vi "move and read QPD.vi"(7 "new position":dbl, 8 "error in":errorcluster, 10 "handle in":i32, 11 "data":dbl[](array[numeric]) format="%0.2f") -> (0 "error out":errorcluster, 2 "handle out":i32, 4 "QPD SD":dbl, 5 "position out":dbl, 6 "QPD mean":dbl)   [LabVIEW 2019]
uses:
  <vilib>/Analysis/NI_AALBase.lvlib
  controller/SubVIs_nanostage/Madlib.dll
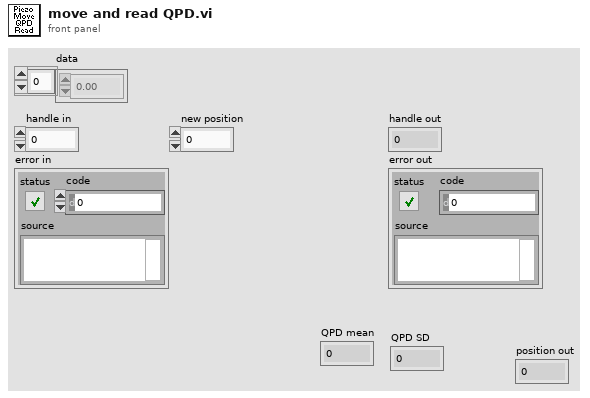
[diagram p1: front panel]
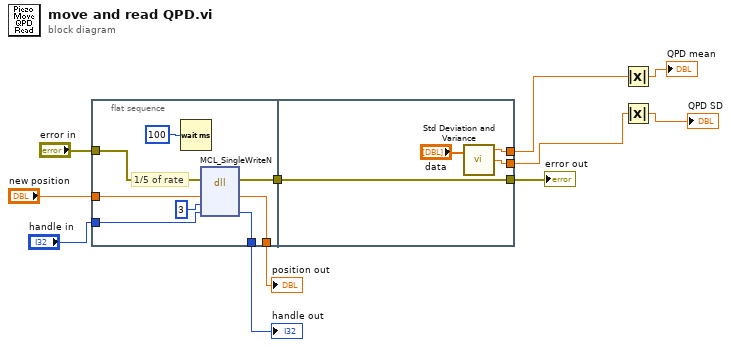
[diagram p0: block diagram]
diagram:
  n1 = flat-sequence {
    tunnel: "handle in" -> [w18]
    tunnel: [w14] -> w11
    tunnel: [w16] -> w9
    tunnel: "error in" -> [w19]
    tunnel: [w15] -> w7
    tunnel: "new position" -> [w13]
    tunnel: w7 -> [w20]
    tunnel: [w20] -> w5
    tunnel: [w23] -> w4
    tunnel: [w22] -> w2
    frame #0 {
      # "1/5 of rate"
      n2 = Wait (ms)(milliseconds to wait=u32 100) -> ()  [unwired: 1 out]
      n3 = dll-call lib="C:/Users/admin/Desktop/controller/SubVIs_nanostage/MADLib.dll" fn="MCL_SingleWriteN"(error in=w19, "position"=w13, "axis"=3, "handle"=w18) -> (error out=w15:errorcluster, "position"=w14:dbl, "handle"=w16:i32)  [unwired: 4 in, 1 out]
    }
    frame #1 {
      n4 = call <vilib>:"Std Deviation and Variance.vi"("X"="data") -> ("mean"=w23:dbl, "standard deviation"=w22:dbl)  [unwired: 1 in, 1 out]
    }
  }
  n5 = Absolute Value(x=w4) -> (abs(x)=→"QPD mean":dbl)
  n6 = Absolute Value(x=w2) -> (abs(x)=→"QPD SD":dbl)
  "position out" <- w11
  "handle out" <- w9
  "error out" <- w5
